vi "LV SCISDK Get Parameter Double.vi"(8 "error in (no error)":errorcluster, 10 "handle":u64, 11 "Path":string) -> (0 "error out":errorcluster, 1 "function return":i32, 2 "handle out":u64, 3 "value":dbl)   [LabVIEW 2021, in "SciSDK_Labview.lvlib"]
doc: "You need this VI to call native dll method to get a double parameter value"
uses:
  SciSDK_Labview.lvlib
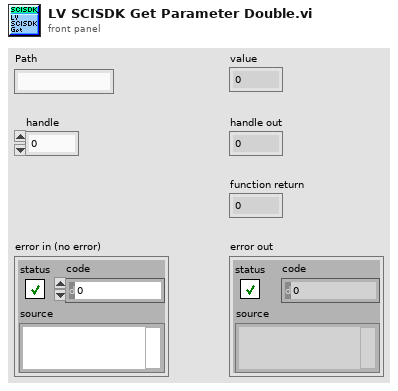
[diagram p1: front panel]
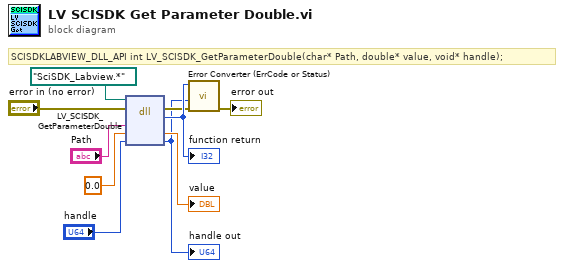
[diagram p0: block diagram]
diagram:
  # "SCISDKLABVIEW_DLL_API int LV_SCISDK_GetParameterDouble(char* Path, double* value, void* handle);"
  n1 = dll-call lib="C:/git/scisdk/SciSDK_VC++/x64/Debug/SciSDK_Labview.dll" fn="LV_SCISDK_GetParameterDouble"(path in=path "SciSDK_Labview.*", error in="error in (no error)", "Path"="Path", "value"=0.0, "handle"="handle") -> (error out=w4:errorcluster, "return type"=w10:i32, "value"=→"value":dbl, "handle"=w1:u64)  [unwired: 2 in, 1 out]
  "function return" <- w10
  "handle out" <- w1
  n2 = call "Error Converter (ErrCode or Status).vi"("error in (no error)"=w4, "handle"=w1, "error code"=w10) -> ("error out"=→"error out":errorcluster)  [unwired: 8 in]
